vi "setSizeAdjustPolicy.vi"(8 "Error In":errorcluster, 10 "policy":T1 items=["AdjustIgnored", "AdjustToContentsOnFirstShow", "AdjustToContents"], 11 "QAbstractScrollArea In":refnum<class "QAbstractScrollArea.lvclass">) -> (0 "Error Out":errorcluster, 3 "QAbstractScrollArea Out":refnum<class "QAbstractScrollArea.lvclass">)   [LabVIEW 2014, in "QAbstractScrollArea.lvclass"]
doc: "LabVIEW-specific documentation is not yet available. See <b>http://doc.qt.io/qt-5/QAbstractScrollArea.html#setSizeAdjustPolicy</b>"
uses:
  QAbstractScrollArea.lvclass
  SizeAdjustPolicy.ctl
  LQ Core/LQIdentity/LQIdentity.lvclass/LQIdentity.ctl
  LQ Core/LQ Core.lvlib
  LQ Core/LQIdentity/LQIdentity.lvclass
panel:
  # "Copyright (c) 2016 Sze Howe Koh\n\nThis Source Code Form is subject to the terms of the Mozilla Public\nLicense, v. 2.0. If a copy of the MPL was not distributed with this\nfile, You can obtain one at http://mozilla.org/MPL/2.0/."
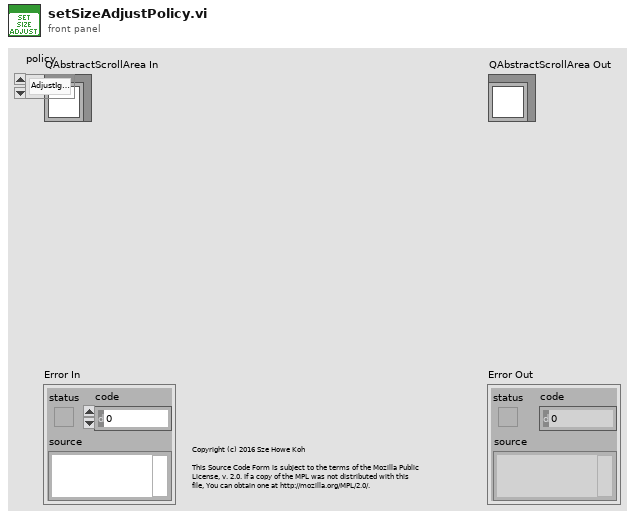
[diagram p1: front panel]
types:
  T1 = typedef "QAbstractScrollArea.lvclass/SizeAdjustPolicy.ctl" = i32
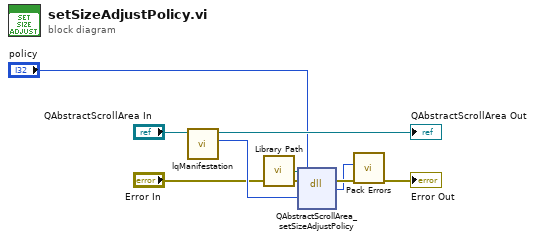
[diagram p0: block diagram]
diagram:
  n1 = call "lqManifestation.vi"("LQIdentity in"="QAbstractScrollArea In") -> ("Manifestation"=w6:u64, "LQIdentity out"=→"QAbstractScrollArea Out":refnum<class "QAbstractScrollArea.lvclass">)  [unwired: 9 in]
  n2 = call "Library Path.vi"() -> ("Library Path"=w7:path)
  n3 = dll-call lib="?" fn="QAbstractScrollArea_setSizeAdjustPolicy"(path in=w7, error in="Error In", "_instance"=w6, "policy"="policy") -> (error out=w4:errorcluster, w2:i32)  [unwired: 3 in, 1 out]
  n4 = call "Pack Errors.vi"("Error In"=w4, "Error Code"=w2) -> ("Error Out"=→"Error Out":errorcluster)  [unwired: 9 in]
